vi "LoadWaveform (subVI).vi"(0 "Axis":u32, 1 "Number of Position Values (steps)":u32=2 min=2 max=1000, 2 "DAC Rate (ms)  (time between steps)":dbl=0.0333333 min=0.0333333 max=5.0 format="%.4f", 3 "Input Data Array":dbl[](array[numeric]) format="%.2f", 4 "Handle":i32) -> (5 "Return Code":i32)   [LabVIEW 2012]
uses:
  Madlib.dll
panel:
  out "?":string
  # "This is an example of loading and triggering a position control \nwaveform in a single step."
  # "X = 1\nY = 2\nZ = 3"
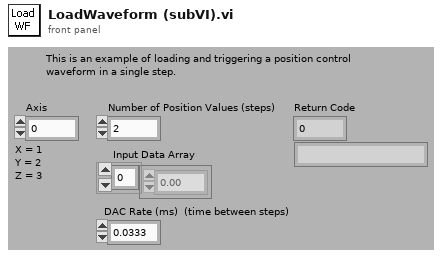
[diagram p1: front panel]
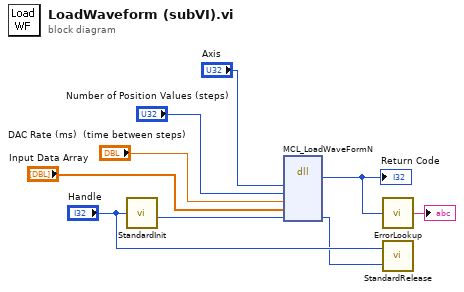
[diagram p0: block diagram]
diagram:
  n1 = call "StandardInit.vi"("Incoming Handle"="Handle") -> ("Outgoing Handle"=w8:i32)
  n2 = dll-call lib="C:/Users/Labview/Desktop/SRR/Madlib_x64/Labview Examples/MADLib.dll" fn="MCL_LoadWaveFormN"("axis"="Axis", "DataPoints"="Number of Position Values (steps)", "milliseconds"="DAC Rate (ms)  (time between steps)", "waveform"="Input Data Array", "handle"=w8) -> (w2:i32, "handle"=w3:i32)  [unwired: 7 in, 2 out]
  "Return Code" <- w2
  n3 = call "ErrorLookup.vi"("Error Code"=w2) -> ("Error"=→"?":string)
  n4 = call "StandardRelease.vi"("Outgoing Handle"=w3, "Incoming Handle"="Handle") -> ()  [unwired: 1 in]
